vi "valves.vi"() -> ()   [LabVIEW 2016]
panel:
  in  "TBA":bool[](array[boolean])
  in  "Pump Valve":bool[](array[boolean])
  in  "Gate Valve":bool[](array[boolean])
  in  "Roughing Valve":bool[](array[boolean])
  # "Turbo Pump"
  # "Scroll (Roughing) Pump"
  # "Back\nPressure\nReadout"
  # "Chamber\nPressure\nReadout"
  # "Chamber"
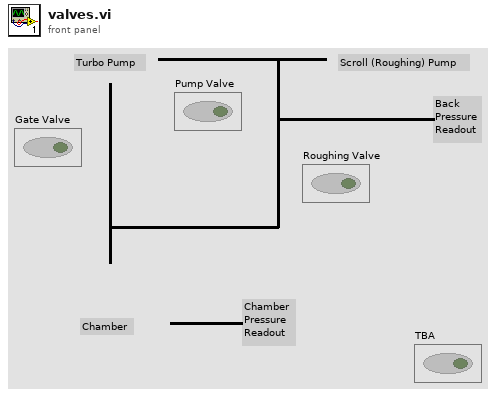
[diagram p1: front panel]
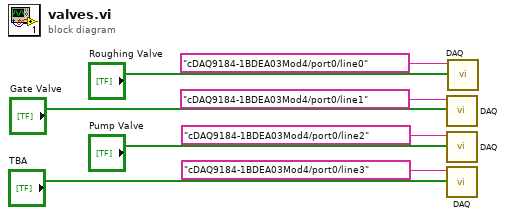
[diagram p0: block diagram]
diagram:
  n1 = call "DAQ.vi"(8:"Gate Valve", 11:tag "cDAQ9184-1BDEA03Mod4/port0/line1" ("lines")) -> ()  [unwired: 10 in]
  n2 = call "DAQ.vi"(8:"Pump Valve", 11:tag "cDAQ9184-1BDEA03Mod4/port0/line2" ("lines")) -> ()  [unwired: 10 in]
  n3 = call "DAQ.vi"(8:"TBA", 11:tag "cDAQ9184-1BDEA03Mod4/port0/line3" ("lines")) -> ()  [unwired: 10 in]
  n4 = call "DAQ.vi"(8:"Roughing Valve", 11:tag "cDAQ9184-1BDEA03Mod4/port0/line0" ("lines")) -> ()  [unwired: 10 in]
